vi "solar_msg Q HS.vi"(8 "error in (no error)":errorcluster, 9 "TLM_DATA":variant, 10 "TLM":string, 11 "CMD_DATA ('HS' Attr)":variant) -> (0 "error out":errorcluster)   [LabVIEW 2018]
doc: "This returns telemetry to the handshake queue specified as the <b>CMD_DATA</b> 'HS' variant attribute. If an error exists it is returned in the <b>TLM_DATA</b> 'ERROR' variant attribute."
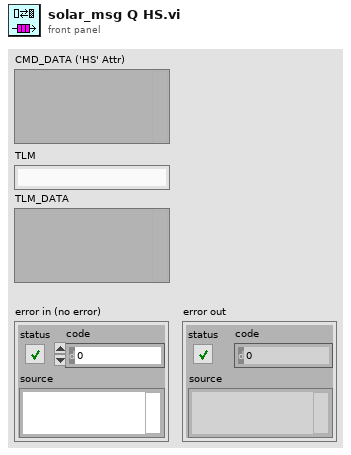
[diagram p1: front panel]
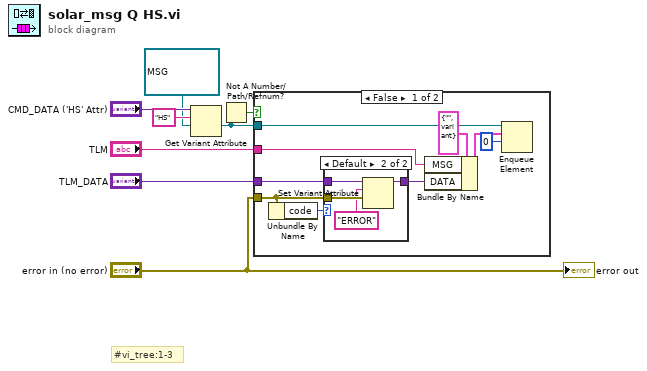
[diagram p0: block diagram]
diagram:
  # "#vi_tree:1-3"
  n1 = Get Variant Attribute(Variant="CMD_DATA ('HS' Attr)", name="HS", default value (empty Variant)=refnum<queue> refnum ("Queue in")) -> (value=w2:refnum<queue>)  [unwired: 1 in, 3 out]
  n2 = Not A Number/Path/Refnum?(number/path/refnum=w2) -> (NaN/Path/Refnum?=w5:bool)
  n3 = case shown="False" w5 {
    tunnel: w2 -> [w17 _]
    tunnel: "error in (no error)" -> [w15 _]
    tunnel: "TLM_DATA" -> [w10 _]
    tunnel: "TLM" -> [w9 _]
    frame False {
      n4 = Unbundle By Name(w15) -> ("code"=w14:i32)
      n5 = case shown="Default" w14 {
        tunnel: w15 -> [_ w22]
        tunnel: [w18 w20] -> w11
        tunnel: w10 -> [w18 w19]
        frame 0 {
        }
        frame Default {
          n6 = Set Variant Attribute(Variant=w19, name="ERROR", value=w22) -> (Variant out=w20:variant)  [unwired: 1 in, 2 out]
        }
      }
      n7 = Bundle By Name(cluster=cluster{"MSG":string, "DATA":variant} {"MSG"="", "DATA"=variant} ("MSG"), "MSG"=w9, "DATA"=w11) -> (w12:cluster{"MSG":string, "DATA":variant})
      n8 = Enqueue Element(queue=w17, element=w12, timeout in ms (-1)=0) -> ()  [unwired: 1 in, 3 out]
    }
    frame True {
    }
  }
  "error out" <- "error in (no error)"
